vi "ScanAction.vi"(8 "error in (no error)":errorcluster caption="entrée d'erreur (pas d'erreur)", 9 "IndicePoint":i32, 10 "Dir":bool, 11 "Tools In":refnum<class "YokoGS200.lvclass"> caption="DNL_LabVIEW Object in") -> (0 "error out":errorcluster caption="sortie d'erreur", 2 "ScanParsOut":dbl[](array[numeric]), 3 "Tools Out":refnum<class "YokoGS200.lvclass"> caption="DNL_LabVIEW Object out")   [LabVIEW 2019, in "YokoGS200.lvclass"]
uses:
  YokoGS200.lvclass
  C:/Programmes Labview/LabScanV1A/DevicesClass/BaseDevice/BaseDevice.lvclass
  YokoGS200.lvclass/YokoGS200.ctl
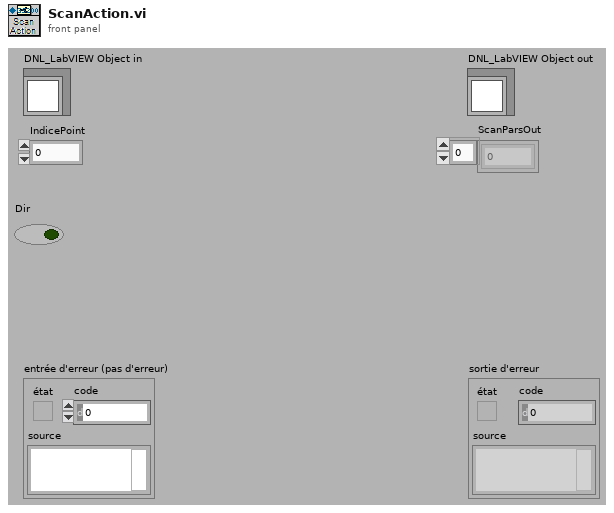
[diagram p1: front panel]
types:
  T1 = typedef "YokoGS200.lvclass/YokoGS200_Func.ctl" = enum16{"SetVoltage (V)", "SetCurrent (A)"}
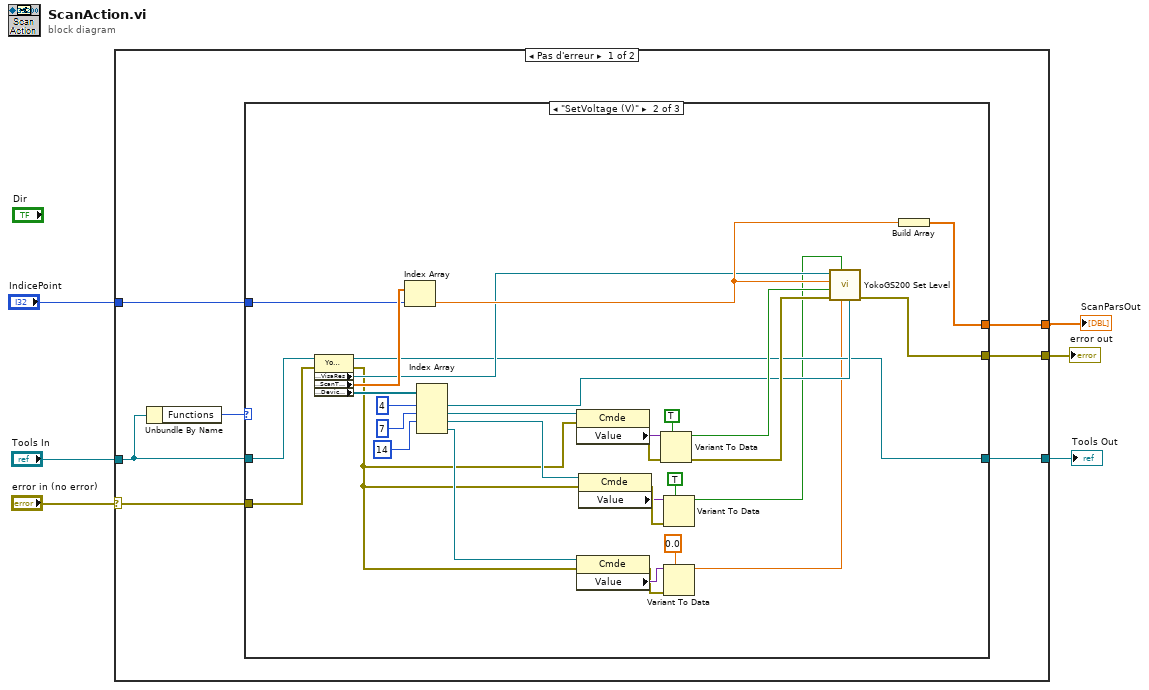
[diagram p0: block diagram]
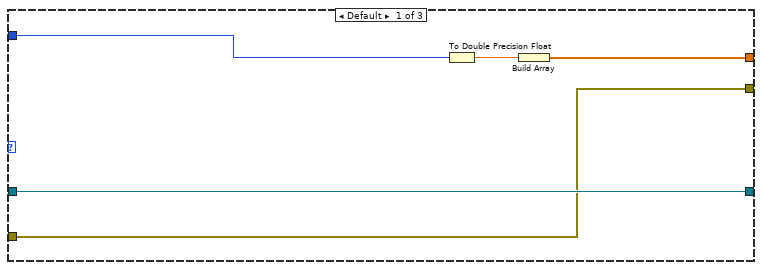
[diagram p2: hidden frame]
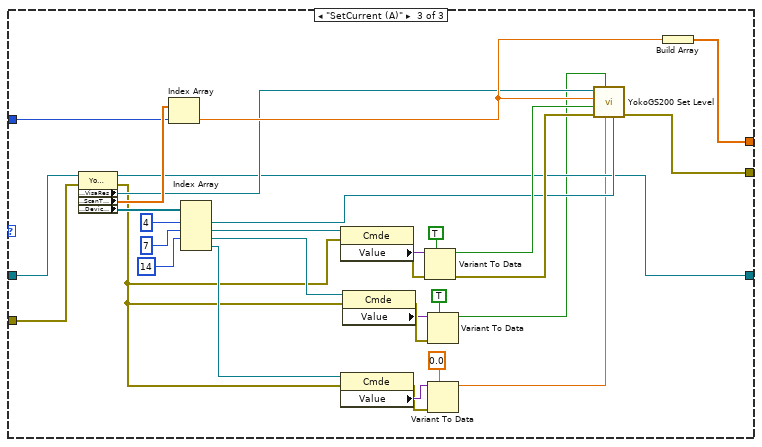
[diagram p3: hidden frame]
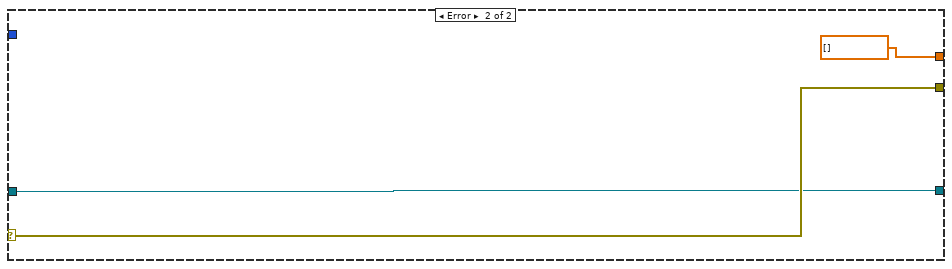
[diagram p4: hidden frame]
diagram:
  n1 = case shown="Pas d'erreur" "error in (no error)" {
    selector: "error in (no error)" -> [w10 w83]
    tunnel: "Tools In" -> [w11 w82]
    tunnel: [w9 dbl[] []] -> w1
    tunnel: [w8 w83] -> w4
    tunnel: [w7 w82] -> w3
    tunnel: "IndicePoint" -> [w12 _]
    frame No Error {
      n2 = Unbundle By Name(w11) -> ("Functions"=w13:T1)
      n3 = case shown="\"SetVoltage (V)\"" w13 {
        tunnel: [w14 w46 w77] -> w9
        tunnel: w12 -> [w18 w24 w55]
        tunnel: [w16 w32 w63] -> w7
        tunnel: w11 -> [w16 w49 w80]
        tunnel: w10 -> [w15 w48 w79]
        tunnel: [w15 w19 w50] -> w8
        frame Default {
          n4 = To Double Precision Float(number=w18) -> (double precision float=w17:dbl)
          n5 = Build Array(w17) -> (w14:dbl[])
        }
        frame "SetVoltage (V)" {
          n6 = property class="YokoGS200.lvclass"(reference=w49, error in=w48) -> (reference out=w32:refnum<class "YokoGS200.lvclass">, error out=w25:errorcluster, "Accessor:VisaRes"=w36:refnum<visa-resource-name>, "Accessor:ScanTable"=w47:dbl[], "Accessor:DeviceCtrl"=w45:refnum<vi>[])
          n7 = Index Array(array=w47, index=w24) -> (element=w38:dbl)
          n8 = Index Array(array=w45, index #1=4 ("index"), index #2=7 ("index"), index #3=14 ("index")) -> (element #1=w35:refnum<vi>, element #2=w42:refnum<vi>, element #3=w28:refnum<vi>, element #4=w26:refnum<vi>)  [unwired: 1 in]
          n9 = property class="Cmde"(reference=w42, error in=w25) -> (error out=w33:errorcluster, "Value"=w41:variant)  [unwired: 1 out]
          n10 = property class="Cmde"(reference=w26, error in=w25) -> (error out=w21:errorcluster, "Value"=w23:variant)  [unwired: 1 out]
          n11 = property class="Cmde"(reference=w28, error in=w25) -> (error out=w31:errorcluster, "Value"=w29:variant)  [unwired: 1 out]
          n12 = Variant To Data(error in=w33, type=TRUE, Variant=w41) -> (data=w39:bool, error out=w37:errorcluster)
          n13 = Variant To Data(error in=w31, type=TRUE, Variant=w29) -> (data=w27:bool)  [unwired: 1 out]
          n14 = Variant To Data(error in=w21, type=0.0, Variant=w23) -> (data=w20:dbl)  [unwired: 1 out]
          n15 = call <userlib>:"YokoGS200 Set Level.vi"("CtrlRef"=w35, "RampRate(Unit/s)"=w20, "Ramp"=w27, "error in (no error)"=w37, "Auto Range"=w39, "Output Level"=w38, "VISA Rsrc"=w36) -> ("error out"=w19:errorcluster)  [unwired: 3 in, 1 out]
          n16 = Build Array(w38) -> (w46:dbl[])
        }
        frame "SetCurrent (A)" {
          n17 = property class="YokoGS200.lvclass"(reference=w80, error in=w79) -> (reference out=w63:refnum<class "YokoGS200.lvclass">, error out=w56:errorcluster, "Accessor:VisaRes"=w67:refnum<visa-resource-name>, "Accessor:ScanTable"=w78:dbl[], "Accessor:DeviceCtrl"=w76:refnum<vi>[])
          n18 = Index Array(array=w78, index=w55) -> (element=w69:dbl)
          n19 = Index Array(array=w76, index #1=4 ("index"), index #2=7 ("index"), index #3=14 ("index")) -> (element #1=w66:refnum<vi>, element #2=w73:refnum<vi>, element #3=w59:refnum<vi>, element #4=w57:refnum<vi>)  [unwired: 1 in]
          n20 = property class="Cmde"(reference=w73, error in=w56) -> (error out=w64:errorcluster, "Value"=w72:variant)  [unwired: 1 out]
          n21 = property class="Cmde"(reference=w57, error in=w56) -> (error out=w52:errorcluster, "Value"=w54:variant)  [unwired: 1 out]
          n22 = property class="Cmde"(reference=w59, error in=w56) -> (error out=w62:errorcluster, "Value"=w60:variant)  [unwired: 1 out]
          n23 = Variant To Data(error in=w64, type=TRUE, Variant=w72) -> (data=w70:bool, error out=w68:errorcluster)
          n24 = Variant To Data(error in=w62, type=TRUE, Variant=w60) -> (data=w58:bool)  [unwired: 1 out]
          n25 = Variant To Data(error in=w52, type=0.0, Variant=w54) -> (data=w51:dbl)  [unwired: 1 out]
          n26 = call <userlib>:"YokoGS200 Set Level.vi"("CtrlRef"=w66, "RampRate(Unit/s)"=w51, "Ramp"=w58, "error in (no error)"=w68, "Auto Range"=w70, "Output Level"=w69, "VISA Rsrc"=w67) -> ("error out"=w50:errorcluster)  [unwired: 3 in, 1 out]
          n27 = Build Array(w69) -> (w77:dbl[])
        }
      }
    }
    frame Error {
    }
  }
  "error out" <- w4
  "Tools Out" <- w3
  "ScanParsOut" <- w1
